vi "Convert to combo box.vi"(8 "error in (no error)":errorcluster caption="错误输入（无错误）", 10 "CmbBox Ref":refnum<vi>, 11 "Dictionary In":refnum<class "Dictionary.lvclass"> caption="DNL_LabVIEW Object in") -> (0 "error out":errorcluster caption="错误输出", 3 "Dictionary Out":refnum<class "Dictionary.lvclass"> caption="DNL_LabVIEW Object out")   [LabVIEW 2012, in "Dictionary.lvclass"]
uses:
  Dictionary.lvclass
  Dictionary.lvclass/Dictionary.ctl
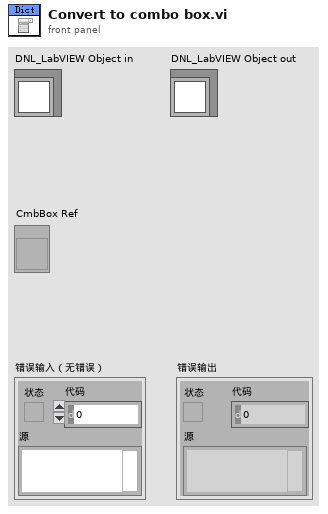
[diagram p1: front panel]
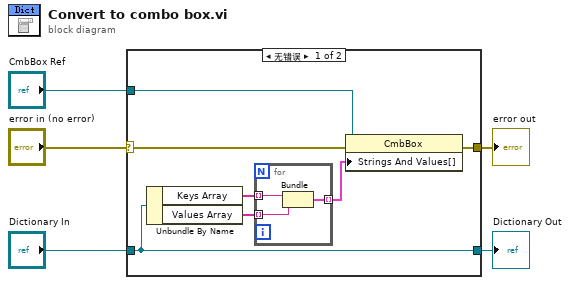
[diagram p0: block diagram]
diagram:
  n1 = case shown="无错误" "error in (no error)" {
    selector: "error in (no error)" -> [w9 w17]
    tunnel: [w7 w17] -> w4
    tunnel: [w12 w16] -> w2
    tunnel: "Dictionary In" -> [w12 w16]
    tunnel: "CmbBox Ref" -> [w6 _]
    frame No Error {
      n2 = Unbundle By Name(w12) -> ("Keys Array"=w11:string[], "Values Array"=w10:string[])
      n3 = for {
        tunnel: w11 -> [w14] mode=indexing
        tunnel: w10 -> [w15] mode=indexing
        tunnel: [w13] -> w8 mode=indexing
        n4 = Bundle("String"=w14, "String"=w15) -> (w13:cluster{"String":string, "String":string})  [unwired: 1 in]
      }
      n5 = property class="CmbBox"(reference=w6, error in=w9, "Strings And Values[]"=w8) -> (error out=w7:errorcluster)  [unwired: 1 out]
    }
    frame Error {
    }
  }
  "error out" <- w4
  "Dictionary Out" <- w2
